vi "check if within limits.vi"(8 "error in (no error)":errorcluster, 10 "Numeric":dbl, 11 "focus in":refnum<class "focus.lvclass">) -> (0 "error out":errorcluster, 1 "coerced?":bool, 2 "approved position":dbl, 3 "focus out":refnum<class "focus.lvclass">)   [LabVIEW 2012, in "focus.lvclass"]
uses:
  focus.lvclass
  focus.lvclass/focus.ctl
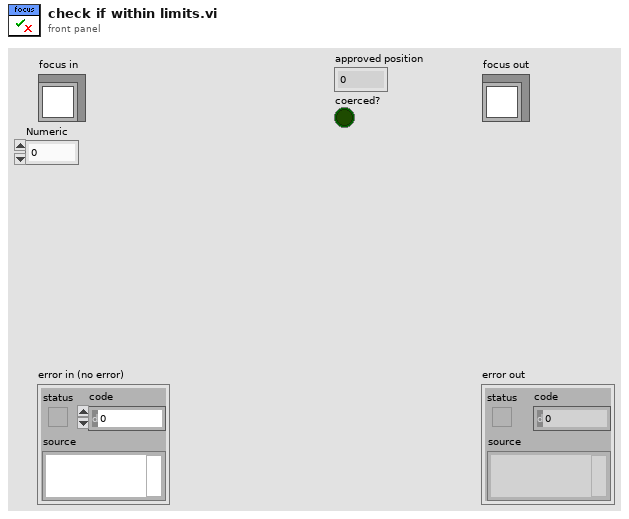
[diagram p1: front panel]
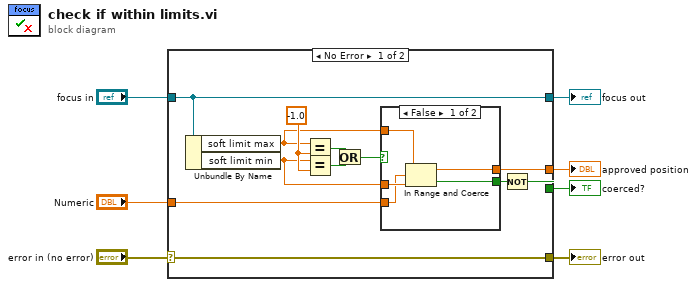
[diagram p0: block diagram]
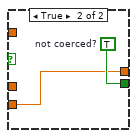
[diagram p2: hidden frame]
diagram:
  n1 = case shown="No Error" "error in (no error)" {
    selector: "error in (no error)" -> [w19 w28]
    tunnel: [w19 w28] -> w6
    tunnel: [w18 w27] -> w4
    tunnel: "focus in" -> [w18 w27]
    tunnel: "Numeric" -> [w11 _]
    tunnel: [w10 _] -> w2
    tunnel: [w8 _] -> w1
    frame No Error {
      w15 = -1.0 ("y")
      n2 = Unbundle By Name(w18) -> ("soft limit max"=w13:dbl, "soft limit min"=w12:dbl)
      n3 = Equal?(x=w13, y=w15) -> (x = y?=w17:bool)
      n4 = Equal?(x=w12, y=w15) -> (x = y?=w16:bool)
      n5 = Or(x=w17, y=w16) -> (x .or. y?=w14:bool)
      n6 = case shown="False" w14 {
        tunnel: [w20 w26] -> w9
        tunnel: w13 -> [w24 _]
        tunnel: w12 -> [w23 _]
        tunnel: w11 -> [w22 w25]
        tunnel: [w21 w25] -> w10
        frame False {
          n7 = In Range and Coerce(upper limit=w24, x=w22, lower limit=w23) -> (coerced(x)=w21:dbl, In Range?=w20:bool)
        }
        frame True {
          w26 = TRUE  # not coerced?
        }
      }
      n8 = Not(x=w9) -> (.not. x?=w8:bool)
    }
    frame Error {
    }
  }
  "error out" <- w6
  "focus out" <- w4
  "approved position" <- w2
  "coerced?" <- w1
